vi "FTW-Test-JobSequencer-GetNextStep.vi"() -> ()   [LabVIEW 2015]
uses:
  source/actor/JobSequencer/FTW-JobSequencer.lvclass
panel:
  out "Pass":bool
  out "Results":cluster{"Jobs":string[][]}[](array[cluster])
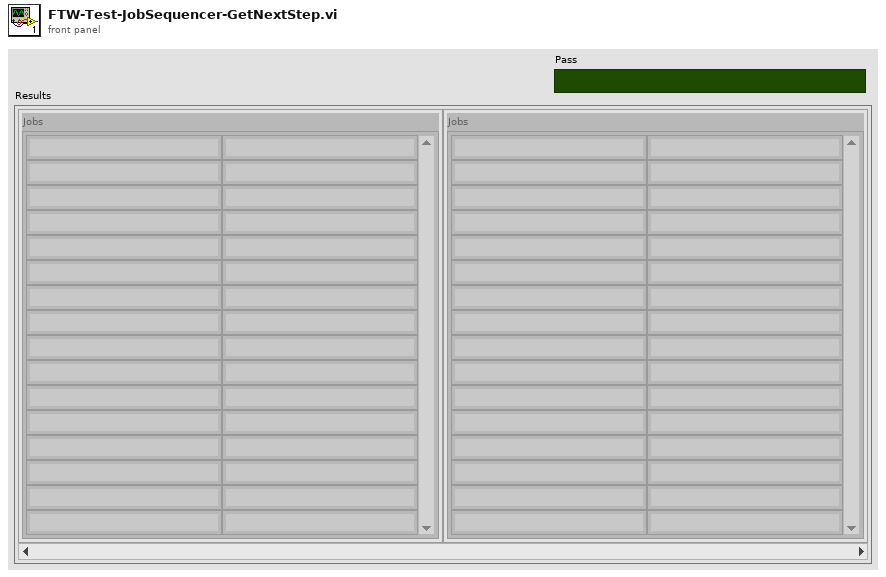
[diagram p1: front panel]
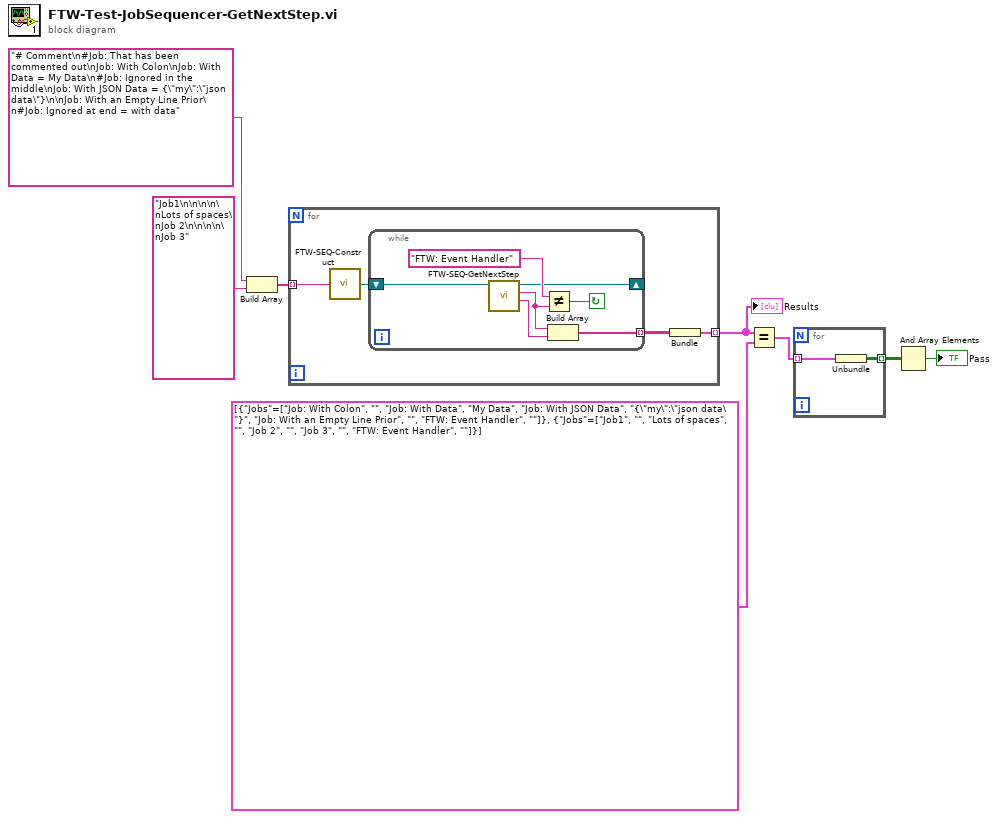
[diagram p0: block diagram]
diagram:
  n1 = Build Array("# Comment\n#Job: That has been commented out\nJob: With Colon\nJob: With Data = My Data\n#Job: Ignored in the middle\nJob: With JSON Data = {\"my\":\"json data\"}\n\nJob: With an Empty Line Prior\n#Job: Ignored at end = with data", "Job1\n\n\n\n\nLots of spaces\nJob 2\n\n\n\n\nJob 3") -> (w7:string[])
  n2 = for {
    tunnel: w7 -> [w11] mode=indexing
    tunnel: [w9] -> w5 mode=indexing
    n3 = call "FTW-SEQ-Construct.vi"("Initial Sequence"=w11) -> ("FTW Job Sequencer"=w12:refnum<class "FTW-JobSequencer.lvclass">)
    n4 = while {
      tunnel: [w15] -> w10 mode=indexing
      shift-right: [w13] -> _
      shift-left: w12 -> [w19]
      stop <- w17 continue-if-true
      n5 = call "FTW-SEQ-GetNextStep.vi"("FTW Job Sequencer"=w19) -> ("Job Data"=w14:string, "Current Job"=w18:string, "FTW Job Sequencer out"=w13:refnum<class "FTW-JobSequencer.lvclass">)  [unwired: 7 in, 1 out]
      n6 = Not Equal?(x="FTW: Event Handler" ("y"), y=w18) -> (x != y?=w17:bool)
      n7 = Build Array(w18, w14) -> (w15:string[])
    }
    n8 = Bundle(w10) -> (w9:cluster{string[][]})  [unwired: 1 in]
  }
  "Results" <- w5
  n9 = Equal?(x=w5, y=cluster{"Jobs":string[][]}[] [{"Jobs"=[["Job: With Colon", ""], ["Job: With Data", "My Data"], ["Job: With JSON Data", "{\"my\":\"json data\"}"], ["Job: With an Empty Line Prior", ""], ["FTW: Event Handler", ""]]}, {"Jobs"=[["Job1", ""], ["Lots of spaces", ""], ["Job 2", ""], ["Job 3", ""], ["FTW: Event Handler", ""]]}] ("Results")) -> (x = y?=w3:cluster{bool[][]}[])
  n10 = for {
    tunnel: w3 -> [w21] mode=indexing
    tunnel: [w20] -> w2 mode=indexing
    n11 = Unbundle(w21) -> (w20:bool[][])
  }
  n12 = And Array Elements(Boolean array=w2) -> (logical AND=→"Pass":bool)
